vi "FTW-WebService-NewRequest.vi"(5 "NI_wsHandle":u32, 7 "httpRequestID":u32, 9 "RequestURI":string) -> (4 "FTW Web Request":refnum<class "FTW-WebService.lvclass">, 15 "error out":errorcluster)   [LabVIEW 2015, in "FTW-WebService.lvclass"]
uses:
  FTW-WebService.lvclass
  Utils/FTW-Web-HTTPResponseCode.ctl
  <vilib>/wsapi/Web Service.lvclass/Web Service.ctl
  <vilib>/wsapi/Web Request.lvclass/Web Request.ctl
  FTW-WebService.lvclass/FTW-WebService.ctl
  <vilib>/wsapi/Web Request.lvclass
  <vilib>/wsapi/Web Service.lvclass
panel:
  # "Inputs"
  # "Outputs"
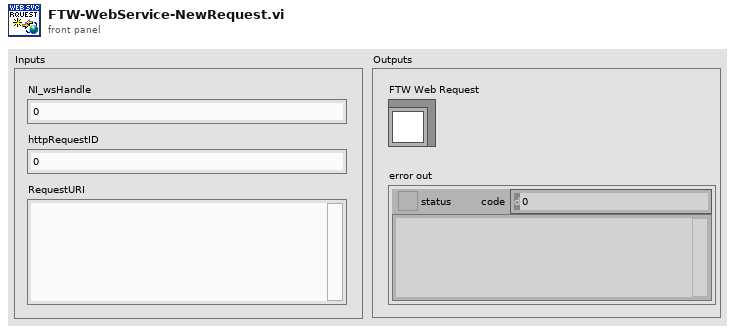
[diagram p1: front panel]
types:
  T1 = typedef "FTW-Web-HTTPResponseCode.ctl" = i32
  T2 = cluster{"HTTP Response Code":T1, "Response Body":string}
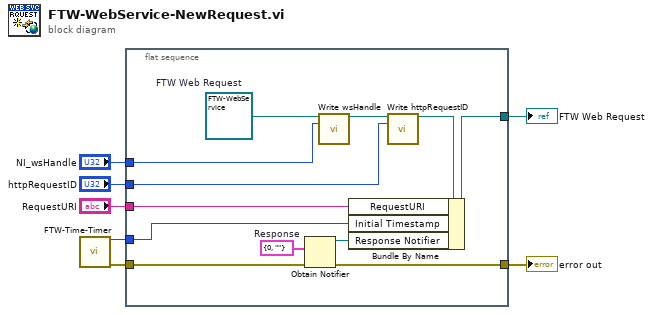
[diagram p0: block diagram]
diagram:
  n1 = call "FTW-Time-Timer.vi"() -> ("Current Tick Count"=w7:u32, "error out"=w1:errorcluster)  [unwired: 13 in, 1 out]
  n2 = flat-sequence {
    tunnel: w7 -> [w12]
    tunnel: [w14] -> w4
    tunnel: "NI_wsHandle" -> [w15]
    tunnel: "httpRequestID" -> [w18]
    tunnel: "RequestURI" -> [w13]
    tunnel: [w9] -> w2
    tunnel: w1 -> [w8]
    frame #0 {
      w10 = T2 {"HTTP Response Code"=0, "Response Body"=""}  # Response
      w17 = refnum<class "FTW-WebService.lvclass"> refnum  # FTW Web Request
      n3 = Obtain Notifier(notification data type=w10, error in (no error)=w8) -> (notifier out=w11:refnum<notifier>, error out=w9:errorcluster)  [unwired: 2 in, 1 out]
      n4 = call <vilib>:"Write wsHandle.vi"("NI_Web Service in"=w17, "wsHandle"=w15) -> ("NI_Web Service out"=w16:refnum<class "FTW-WebService.lvclass">)  [unwired: 13 in]
      n5 = call <vilib>:"Write httpRequestID.vi"("NI_Web Request in"=w16, "httpRequestID"=w18) -> ("NI_Web Request out"=w19:refnum<class "FTW-WebService.lvclass">)  [unwired: 13 in]
      n6 = Bundle By Name(cluster=w19, "RequestURI"=w13, "Initial Timestamp"=w12, "Response Notifier"=w11) -> (w14:refnum<class "FTW-WebService.lvclass">)
    }
  }
  "FTW Web Request" <- w4
  "error out" <- w2
